vi "PRL Access Buffer.vi"(9 "PMU Data Buffers":T1, 10 "Read Data?":bool, 11 "Initialize Buffer?":bool) -> (0 "System Data":sgl[][](array[numeric]), 1 "Digital Values":bool[][](array[boolean]), 2 "Analog Values":sgl[][](array[numeric]), 3 "Phasor Values":csg[][](array[numeric]), 4 "First Buffer Filled":bool, 5 "Timestamp Values":timestamp[](array[timestamp]), 7 "Buffer Full":bool)   [LabVIEW 2017, in "PMU Recorder Light.lvlib"]
uses:
  PMU Recorder Light.lvlib
  Setting Choice.ctl
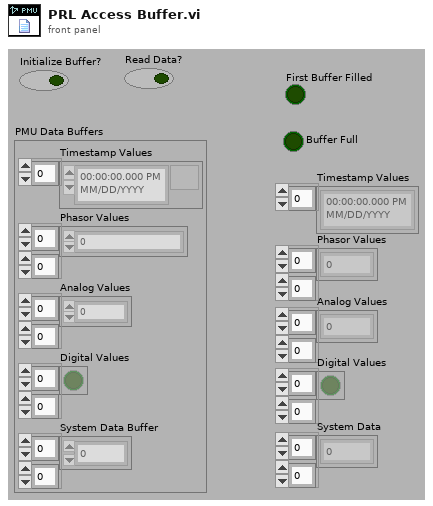
[diagram p1: front panel]
types:
  T1 = cluster{"Timestamp Values":timestamp[], "Phasor Values":csg[][], "Analog Values":sgl[][], "Digital Values":bool[][], "System Data Buffer":sgl[][]}
  T2 = typedef "PMU Recorder Light.lvlib/Setting Choice.ctl" = enum16{"Analog Data Points Allowed Equals", "Complex Data Points Allowed Equals", "Seconds Before Reset After Wait for Config Fails", "Number of Live Buffer in Access Buffer ", "Number of Connection Attempts", "Live Data Buffer Size", "dt Tolerance", "Data Rate History", "ALL"}
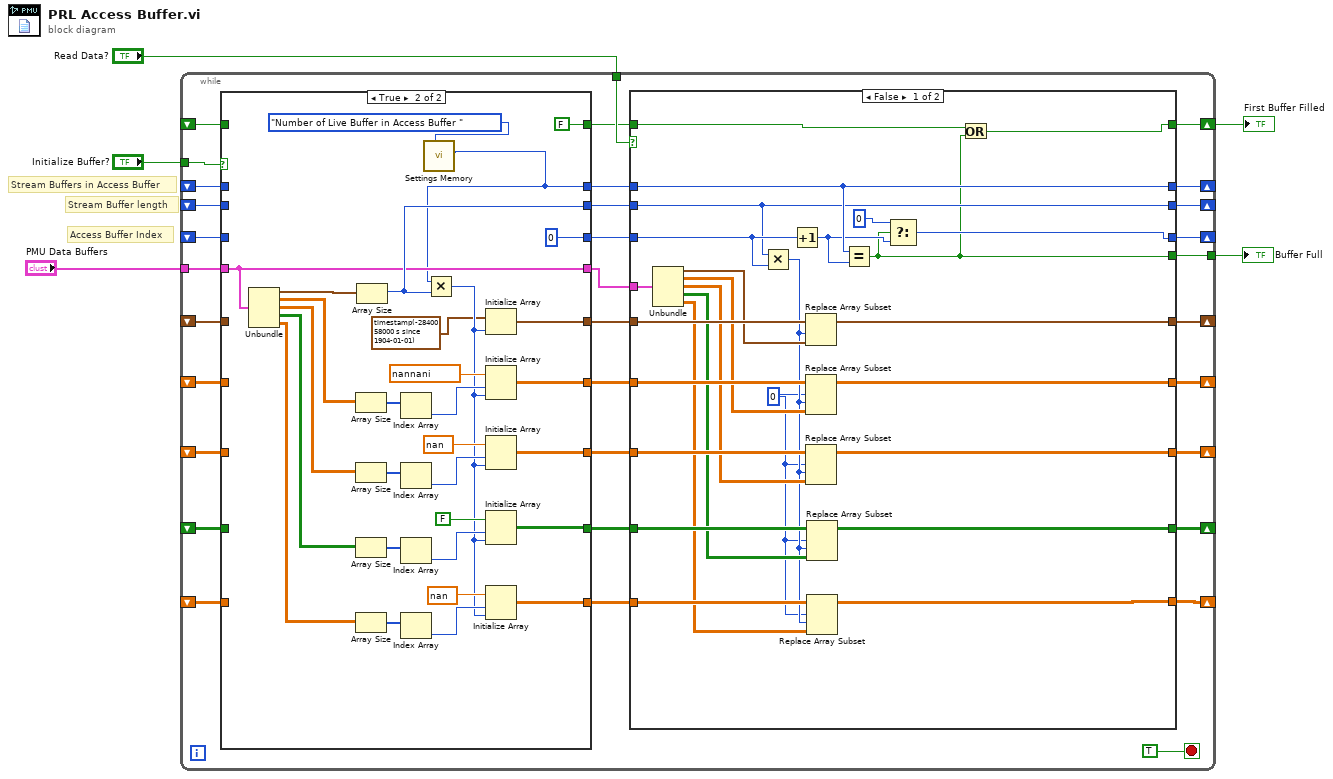
[diagram p0: block diagram]
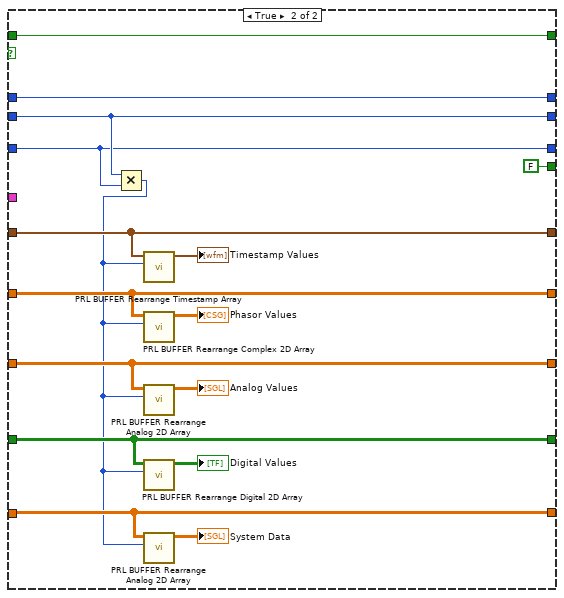
[diagram p2: hidden frame]
diagram:
  # "Access Buffer Index"
  # "Stream Buffer length"
  # "Stream Buffers in Access Buffer"
  n1 = while {
    tunnel: "PMU Data Buffers" -> [w37]
    tunnel: "Initialize Buffer?" -> [w38]
    shift-right: [w19] -> _
    shift-left: _ -> [w34]
    shift-right: [w10] -> _
    shift-left: _ -> [w33]
    shift-right: [w18] -> _
    shift-left: _ -> [w30]
    shift-right: [w17] -> _
    shift-left: _ -> [w25]
    shift-right: [w16] -> _
    shift-left: _ -> [w24]
    shift-right: [w15] -> _
    shift-left: _ -> [w23]
    shift-right: [w14] -> _
    shift-left: _ -> [w22]
    shift-right: [w11] -> _
    shift-left: _ -> [w36]
    tunnel: "Read Data?" -> [w12]
    tunnel: [w9] -> w2
    shift-right: [w7] -> w1
    shift-left: _ -> [w8]
    stop <- TRUE stop-if-true
    n2 = case shown="True" w38 {
      tunnel: w37 -> [w86 w101]
      tunnel: w36 -> [w85 _]
      tunnel: [w90 w108] -> w29
      tunnel: [w89 w107] -> w28
      tunnel: [w88 w106] -> w27
      tunnel: [w87 w105] -> w26
      tunnel: [w91 w104] -> w32
      tunnel: w34 -> [w83 _]
      tunnel: [w83 0 ("Number of Buffers in File Buffer")] -> w21
      tunnel: [w85 w92] -> w20
      tunnel: w33 -> [w84 _]
      tunnel: [w84 w102] -> w13
      tunnel: [w86 w101] -> w31
      tunnel: w30 -> [w91 _]
      tunnel: w25 -> [w90 _]
      tunnel: w24 -> [w89 _]
      tunnel: w23 -> [w88 _]
      tunnel: w22 -> [w87 _]
      tunnel: w8 -> [w82 _]
      tunnel: [w82 FALSE ("Read Data?")] -> w6
      frame False {
      }
      frame True {
        n3 = Unbundle(w101) -> ("Timestamp Values"=w121:timestamp[], "Phasor Values"=w120:csg[][], "Analog Values"=w115:sgl[][], "Digital Values"=w112:bool[][], "System Data Buffer"=w109:sgl[][])
        n4 = Array Size(array=w120) -> (size(s)=w119:i32[])
        n5 = Array Size(array=w115) -> (size(s)=w116:i32[])
        n6 = Array Size(array=w112) -> (size(s)=w114:i32[])
        n7 = Array Size(array=w109) -> (size(s)=w110:i32[])
        n8 = Array Size(array=w121) -> (size(s)=w102:i32)
        n9 = Index Array(array=w119) -> (element=w118:i32)  [unwired: 1 in]
        n10 = Index Array(array=w116) -> (element=w117:i32)  [unwired: 1 in]
        n11 = Index Array(array=w114) -> (element=w113:i32)  [unwired: 1 in]
        n12 = Index Array(array=w110) -> (element=w111:i32)  [unwired: 1 in]
        n13 = call "Settings Memory.vi"("Setting Choice"=Setting_Choice."Number of Live Buffer in Access Buffer ") -> ("Output Int32"=w92:i32)  [unwired: 8 in, 2 out]
        n14 = Multiply(x=w92, y=w102) -> (x*y=w96:i32)
        n15 = Initialize Array(timestamp(-2840058000 s since 1904-01-01) ("element"), w96) -> (w104:timestamp[])
        n16 = Initialize Array(csg nan+nani ("element"), w118, w96) -> (w108:csg[][])
        n17 = Initialize Array(sgl nan ("element"), w117, w96) -> (w107:sgl[][])
        n18 = Initialize Array(FALSE ("element"), w113, w96) -> (w106:bool[][])
        n19 = Initialize Array(sgl nan ("element"), w111, w96) -> (w105:sgl[][])
      }
    }
    n20 = case shown="False" w12 {
      tunnel: w32 -> [w65 w76]
      tunnel: w31 -> [w64 _]
      tunnel: w29 -> [w62 w74]
      tunnel: w28 -> [w61 w72]
      tunnel: w27 -> [w60 w70]
      tunnel: w26 -> [w59 w68]
      tunnel: w21 -> [w54 w79]
      tunnel: w20 -> [w46 w81]
      tunnel: [w42 w79] -> w19
      tunnel: [w53 w76] -> w18
      tunnel: [w52 w74] -> w17
      tunnel: [w51 w72] -> w16
      tunnel: [w50 w70] -> w15
      tunnel: [w49 w68] -> w14
      tunnel: w13 -> [w45 w80]
      tunnel: [w46 w81] -> w11
      tunnel: [w45 w80] -> w10
      tunnel: [w39 FALSE] -> w9
      tunnel: [w41 w66] -> w7
      tunnel: w6 -> [w40 w66]
      frame False {
        w47 = 0 ("disabled index (col)")
        n21 = Unbundle(w64) -> ("Timestamp Values"=w63:timestamp[], "Phasor Values"=w58:csg[][], "Analog Values"=w57:sgl[][], "Digital Values"=w56:bool[][], "System Data Buffer"=w55:sgl[][])
        n22 = Multiply(x=w45, y=w54) -> (x*y=w48:i32)
        n23 = Increment(x=w54) -> (x+1=w43:i32)
        n24 = Replace Array Subset(array=w65, new element=w63, index=w48) -> (w53:timestamp[])
        n25 = Replace Array Subset(array=w62, new element=w58, index (row)=w47, index (col)=w48) -> (w52:csg[][])
        n26 = Replace Array Subset(array=w61, new element=w57, index (row)=w47, index (col)=w48) -> (w51:sgl[][])
        n27 = Replace Array Subset(array=w60, new element=w56, index (row)=w47, index (col)=w48) -> (w50:bool[][])
        n28 = Replace Array Subset(array=w59, new element=w55, index (row)=w47, index (col)=w48) -> (w49:sgl[][])
        n29 = Equal?(x=w46, y=w43) -> (x = y?=w39:bool)
        n30 = Select(t=0 ("Number of Buffers in File Buffer"), s=w39, f=w43) -> (s? t:f=w42:i32)
        n31 = Or(x=w40, y=w39) -> (x .or. y?=w41:bool)
      }
      frame True {
        n32 = Multiply(x=w80, y=w79) -> (x*y=w67:i32)
        n33 = call "PRL BUFFER Rearrange Timestamp Array.vi"("Cut Index"=w67, "Array In"=w76) -> ("Array Out"=→"Timestamp Values":timestamp[])  [unwired: 9 in]
        n34 = call "PRL BUFFER Rearrange Complex 2D Array.vi"("Cut Index"=w67, "Array In"=w74) -> ("Array Out"=→"Phasor Values":csg[][])  [unwired: 9 in]
        n35 = call "PRL BUFFER Rearrange Analog 2D Array.vi"("Cut Index"=w67, "Array In"=w72) -> ("Array Out"=→"Analog Values":sgl[][])  [unwired: 9 in]
        n36 = call "PRL BUFFER Rearrange Digital 2D Array.vi"("Cut Index"=w67, "Array In"=w70) -> ("Array Out"=→"Digital Values":bool[][])  [unwired: 9 in]
        n37 = call "PRL BUFFER Rearrange Analog 2D Array.vi"("Cut Index"=w67, "Array In"=w68) -> ("Array Out"=→"System Data":sgl[][])  [unwired: 9 in]
      }
    }
  }
  "Buffer Full" <- w2
  "First Buffer Filled" <- w1
